vi "Create File.vi"(9 "File name":string, 10 "Error in":errorcluster) -> (0 "Error code":i32, 2 "file_id":i32, 3 "Error out":errorcluster)   [LabVIEW 2010]
uses:
  Release/HDF5Tools.dll
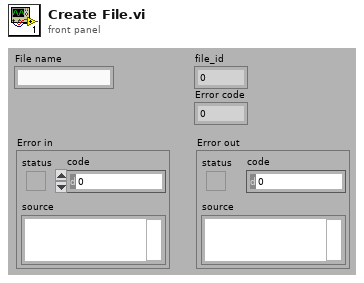
[diagram p1: front panel]
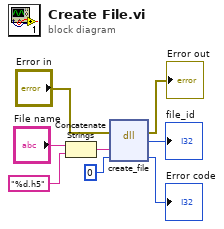
[diagram p0: block diagram]
diagram:
  n1 = Concatenate Strings("File name", "%d.h5" ("name")) -> (w6:string)
  n2 = dll-call lib="Z:/users/alex/projects/HDF5Tools/Release/HDF5Tools.dll" fn="create_file"(error in="Error in", "name"=w6, "error"=0) -> (error out=→"Error out":errorcluster, "file_id"=→"file_id":i32, "error"=→"Error code":i32)  [unwired: 3 in, 1 out]
